vi "10-QNET_MECHKIT_Temperature.vi"() -> ()   [LabVIEW 2012]
doc: "This VI is to be used with the NI-ELVIS and the QNET-Mechatronic Sensors I module. The objective is to calibrate the thermistor to measure the correct temperature."
uses:
  <vilib>/Simulation/Scripting/Companion Diagram/SimConfigNode/SimParams.ctl
  <vilib>/Simulation/Scripting/Companion Diagram/SimConfigNode/_simSolvers.ctl
  <vilib>/Simulation/Implementation/Shared/SIMSCR Execution Mode.ctl
  <vilib>/Simulation/Param Hierarchy/Typedefs/SIMPH Param Control Actions.ctl
  <vilib>/Simulation/Implementation/Shared/NILVSim_ParamChanged.vi
  <vilib>/Simulation/SignalDisplay/Implementation/NILVSim Time Waveform.llb/SIM Time Waveform (scalar).vi
  <vilib>/Simulation/Utility/Implementation/SIM Halt.vi
  <vilib>/Simulation/Implementation/Shared/NILVSim_Manager.vi
  <vilib>/Simulation/Implementation/Shared/NILVSim_FinalizeModel.vi
  <vilib>/Simulation/Implementation/Shared/SIM Unbundle Sim Info.vi
  <vilib>/Utility/error.llb/Clear Errors.vi
  <vilib>/Simulation/Implementation/Shared/NILVSim_GetModelError.vi
  <vilib>/Simulation/Implementation/Shared/SIM Bundle Sim Info.vi
  <vilib>/Simulation/Implementation/Shared/SIMSH Read Queue.vi
  <vilib>/Simulation/Implementation/Shared/NILVSim_Initialize.vi
  <vilib>/DAQmx/read.llb/DAQmx Read.vi
  <vilib>/DAQmx/read.llb/DAQmx Read (Analog DBL 1Chan 1Samp).vi
  <vilib>/Simulation/Utility/Implementation/NILVSim Get Time and IsAcceptedStep.vi
  <vilib>/Simulation/Scripting/Companion Diagram/SimConfigNode/SimDog.xnode
  <vilib>/Simulation/Implementation/XNodeFramework/SimXNode/SimX.xnode
  <vilib>/Simulation/Implementation/Shared/NI_SIM_Implementation.lvlib
panel:
  out "Temperature Sensor (V)":waveform(dbl)(graph)
  out "Temperature (deg C)":dbl(slide) scale=0.0..40.0
  in  "B":dbl
  in  "R0":dbl=47000.0
  out "Temperature Sensor (deg C)":waveform(dbl)(graph)
  in  "T0":dbl=298.0
  in  "Sampling Rate (Hz)":dbl=100.0 min=0.0 max=1000.0 step=25.0 format="%.1f"
  in  "Device":tag="Dev1"
  in  "stop":bool
  # "QNET-MECHKIT Temperature"
  # "NOTE: Place J9 jumper on \"Temperature\" setting."
  # "Measured thermistor resistance is\nR = R0*exp(B*(1/T-1/T0))\nwhere\nR0 is 47 kOhms\nT0 is 298 K\nT is the sensed temperature"
  # "s"
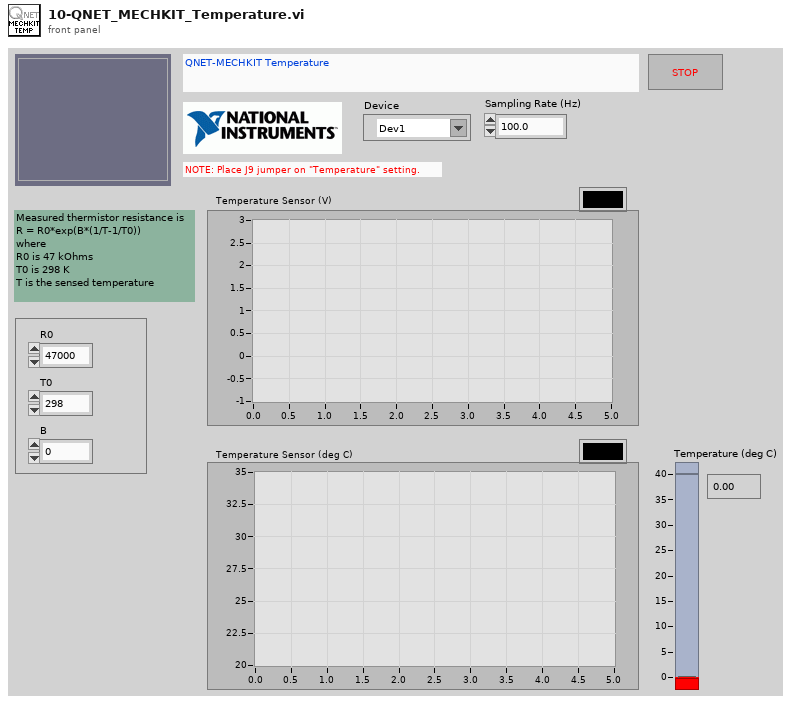
[diagram p1: front panel]
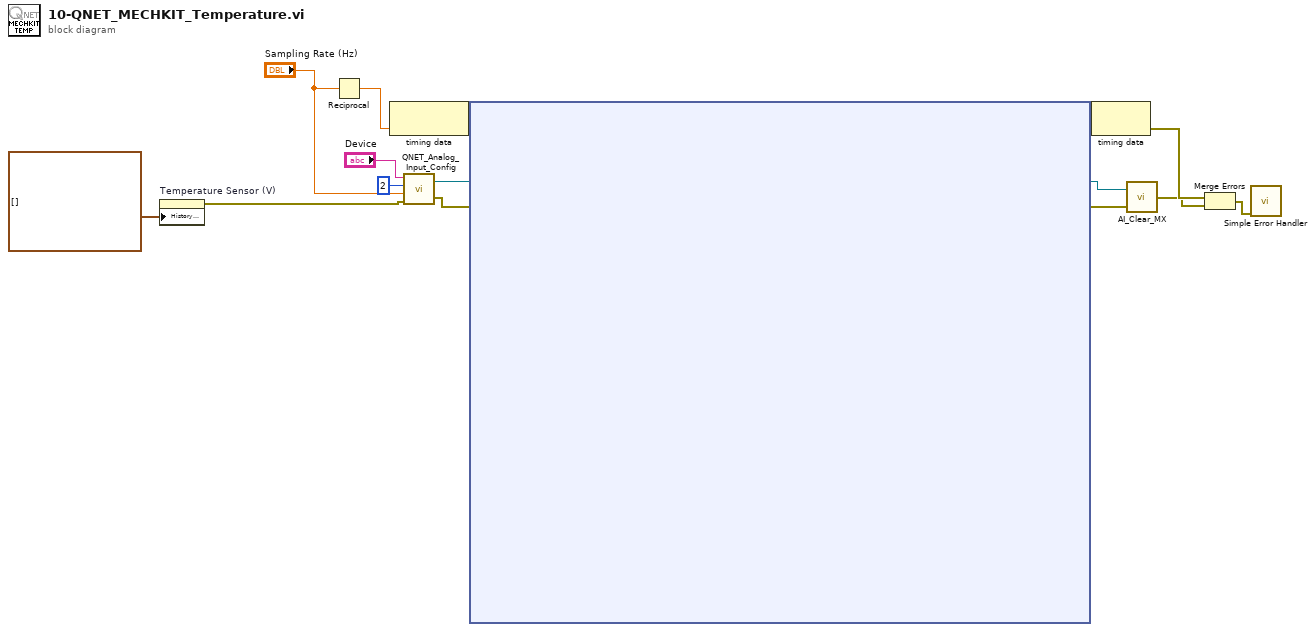
[diagram p0: block diagram]
diagram:
  n1 = property on="Temperature Sensor (V)" class="WFChart (strict)"("History Data"=waveform(dbl)[] []) -> (error out=w3:errorcluster)  [unwired: 2 in, 1 out]
  n2 = Reciprocal(x="Sampling Rate (Hz)") -> (1/x=w1:dbl)
  n3 = node-c288(w1) -> (w14:variant)
  n4 = call "QNET_Analog_Input_Config.vi"("error in"=w3, "sampling rate (Hz)"="Sampling Rate (Hz)", "analog input channel"=u32 2, "dev"="Device") -> ("error out"=w11:errorcluster, "task out"=w10:refnum<k21>)
  n5 = node-c254 ("Simulation Loop")(w14, w11, w10) -> (w13:variant, w9:refnum<k21>, w8:errorcluster)
  n6 = node-c288(w13) -> (w6:errorcluster)
  n7 = call "AI_Clear_MX.vi"("Error in"=w8, "Task in"=w9) -> ("Error out"=w5:errorcluster)
  n8 = Merge Errors(w6, w5) -> (w4:errorcluster)
  n9 = call <vilib>:"Simple Error Handler.vi"("error in (no error)"=w4) -> ()  [unwired: 1 in, 8 out]
